vi "DisplayLiveWindow.vi"(0 "object in":refnum<class "Hamamatsu.lvclass">, 2 "Image Src":T1, 5 "error in (no error)":errorcluster) -> (14 "object out":refnum<class "Hamamatsu.lvclass">, 19 "error out":errorcluster)   [LabVIEW 2021, in "Hamamatsu.lvclass"]
uses:
  Hamamatsu.lvclass
  Hamamatsu.lvclass/Hamamatsu.ctl
  <vilib>/vision/Image Controls.llb/IMAQ Image.ctl
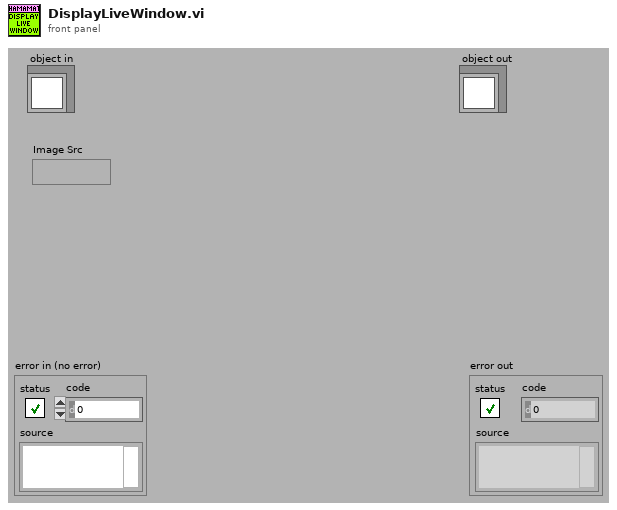
[diagram p1: front panel]
types:
  T1 = typedef "IMAQ Image.ctl" = refnum<image>
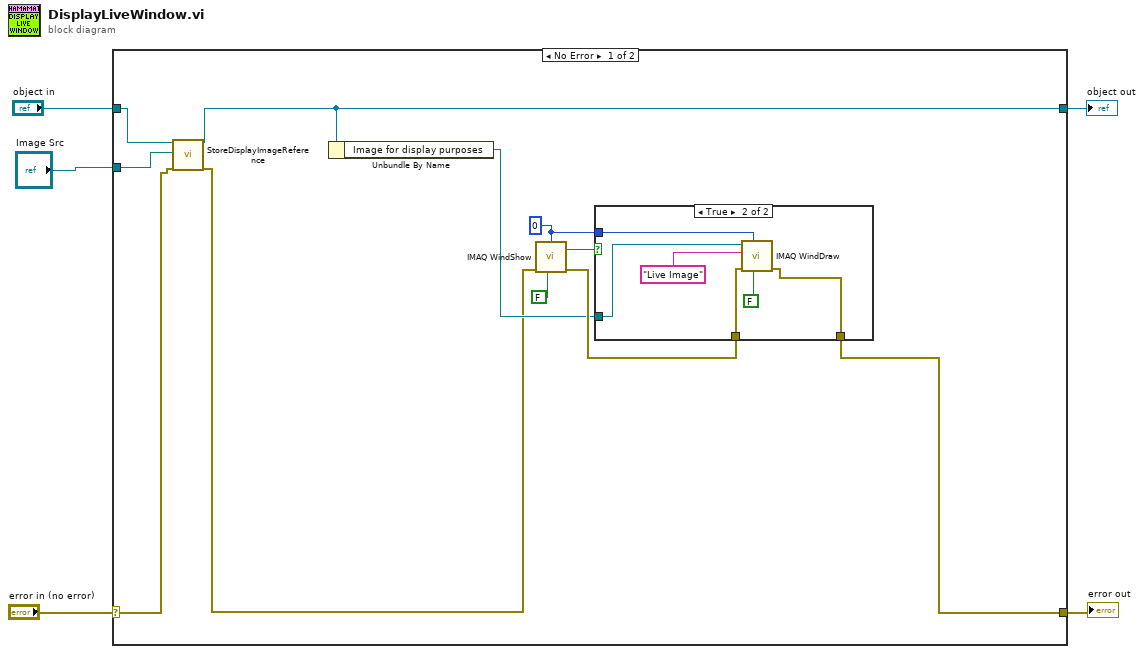
[diagram p0: block diagram]
diagram:
  n1 = case shown="No Error" "error in (no error)" {
    selector: "error in (no error)" -> [w8 w25]
    tunnel: [w11 w25] -> w4
    tunnel: [w10 w24] -> w2
    tunnel: "object in" -> [w9 w24]
    tunnel: "Image Src" -> [w6 _]
    frame No Error {
      w14 = 0 ("Window Number (0...15)")
      n2 = call-dynamic "StoreDisplayImageReference.vi"("object in"=w9, "Image Src"=w6, "error in (no error)"=w8) -> ("object out"=w10:refnum<class "Hamamatsu.lvclass">, "error out"=w7:errorcluster)  [unwired: 14 in, 1 out]
      n3 = Unbundle By Name(w10) -> ("Image for display purposes"=w12:T1)
      n4 = call "IMAQ WindShow"("error in (no error)"=w7, "Get/Set Status? (Set)"=FALSE, "Window Number (0...15)"=w14) -> ("error out"=w15:errorcluster, "Visible?"=w13:bool)  [unwired: 3 in, 1 out]
      n5 = case shown="True" w13 {
        tunnel: w12 -> [_ w21]
        tunnel: w15 -> [w17 w20]
        tunnel: w14 -> [_ w19]
        tunnel: [w17 w18] -> w11
        frame False {
        }
        frame True {
          n6 = call "IMAQ WindDraw"("Resize to Image Size? (Y)"=FALSE, "Window Number (0...15)"=w19, "error in (no error)"=w20, "Title"="Live Image", "Image"=w21) -> ("error out"=w18:errorcluster)  [unwired: 5 in, 1 out]
        }
      }
    }
    frame Error {
    }
  }
  "error out" <- w4
  "object out" <- w2
